vi "aft_Coerce_Word length.vi"(10 "word length in":i32) -> (2 "word length out":u32)   [LabVIEW 2017, in "NI_AdaptiveFilter.lvlib"]
uses:
  <vilib>/addons/Adaptive Filters/NI_AdaptiveFilter.lvlib
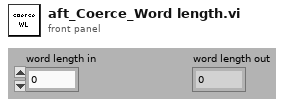
[diagram p1: front panel]
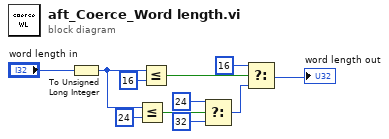
[diagram p0: block diagram]
diagram:
  n1 = To Unsigned Long Integer(number="word length in") -> (unsigned 32bit integer=w7:u32)
  n2 = Less Or Equal?(x=w7, y=24 ("x")) -> (x <= y?=w8:bool)
  n3 = Less Or Equal?(x=w7, y=16 ("x")) -> (x <= y?=w4:bool)
  n4 = Select(t=u32 24 ("x"), s=w8, f=u32 32 ("x")) -> (s? t:f=w11:u32)
  n5 = Select(t=u32 16 ("x"), s=w4, f=w11) -> (s? t:f=→"word length out":u32)
